vi "Detect_Valid_USID.vi"(7 "DUT_USID":u8, 8 "Error In":errorcluster, 10 "Potential_USID_Array":T2[](array[typedef])=[1, 2, 4, 7, 8, 9, 13, 15] max=15, 11 "Semiconductor Module Context":T1) -> (0 "Error Out":errorcluster)   [LabVIEW 2013]
uses:
  Controls/USID.ctl
  <vilib>/NI_TestStand_SemiconductorModule/NI_TestStand_Semiconductor_Module.lvlibp/PinMap/General/SemiconductorModuleContext.ctl
  <vilib>/NI_TestStand_SemiconductorModule/NI_TestStand_Semiconductor_Module.lvlibp/PinMap/General/Publish/PublishDataDoubleFunctionalTest.vi
  <vilib>/NI_TestStand_SemiconductorModule/NI_TestStand_Semiconductor_Module.lvlibp
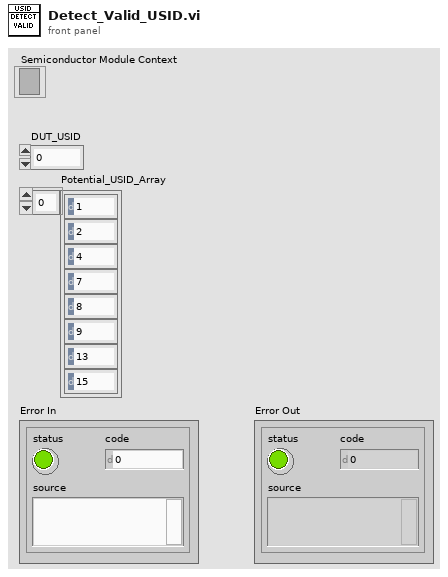
[diagram p1: front panel]
types:
  T1 = typedef "NI_TestStand_Semiconductor_Module.lvlibp/SemiconductorModuleContext.ctl" = refnum<k7>
  T2 = typedef "USID.ctl" = u8
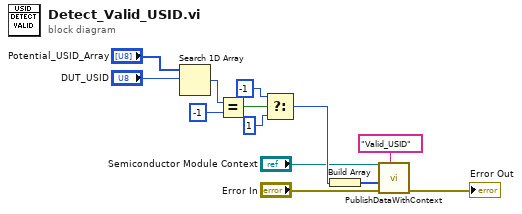
[diagram p0: block diagram]
diagram:
  n1 = Search 1D Array(1D array="Potential_USID_Array", element="DUT_USID") -> (index of element=w9:i32)  [unwired: 1 in]
  n2 = Equal?(x=w9, y=-1) -> (x = y?=w6:bool)
  n3 = Select(t=-1 ("y"), s=w6, f=1 ("y")) -> (s? t:f=w5:i32)
  n4 = Build Array(w5) -> (w10:i32[])
  n5 = call-poly <vilib>:"PublishDataWithContext.vi"("Published Data Id"="Valid_USID", "error in (no error)"="Error In", "Data In"=w10, "Semiconductor Module Context"="Semiconductor Module Context") -> ("error out"=→"Error Out":errorcluster)  [unwired: 6 in, 1 out]
